vi "AIT 1553 - Clear Database.vi"(8 "error in (no error)":errorcluster, 11 "Node Ptr":u64 format="%.0x") -> (0 "error out":errorcluster)   [LabVIEW 2011, in "AIT 1553 Custom Device.lvlib"]
uses:
  AIT 1553 Custom Device.lvlib
  Controls and Global/Global.vi
  <vilib>/NI Veristand/Custom Device Tools/Custom Device Utility Library/NI VeriStand - Search for Item by GUID.vi
  <vilib>/NI Veristand/Custom Device API/Custom Device API.lvlib
  <vilib>/NI Veristand/Custom Device Tools/Custom Device Utility Library/Custom Device Utility Library.lvlib
panel:
  in  "Tag":string
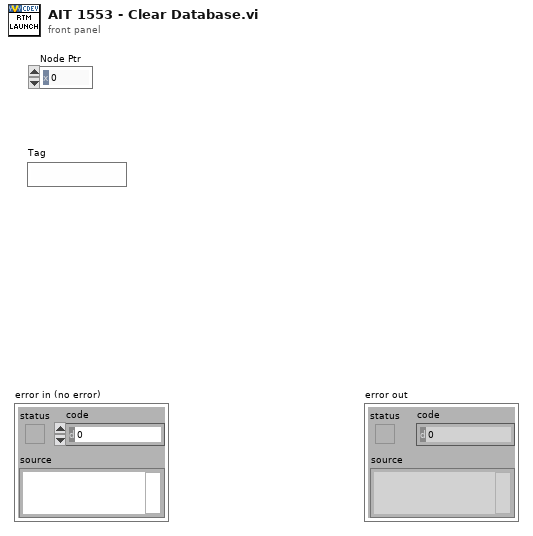
[diagram p1: front panel]
types:
  T1 = typedef "Custom Device API.lvlib/Custom Device Item Ref.ctl" = u64
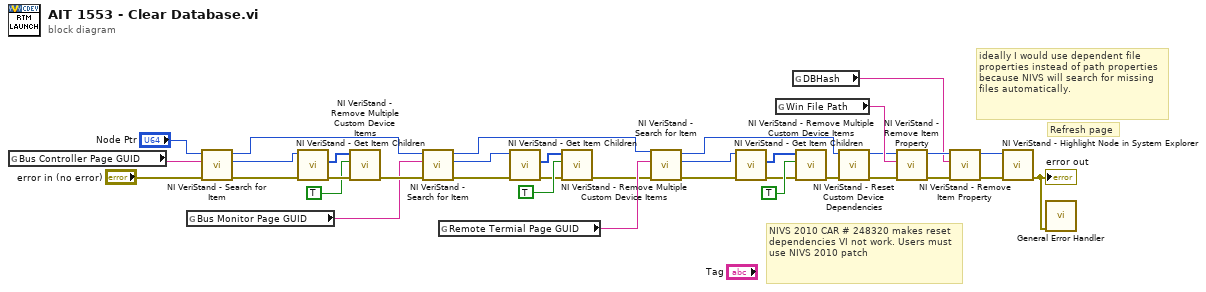
[diagram p0: block diagram]
diagram:
  # "ideally I would use dependent file properties instead of path properties because NIVS will search for missing files automatically."
  # "NIVS 2010 CAR # 248320 makes reset dependencies VI not work. Users must use NIVS 2010 patch"
  # "Refresh page"
  n1 = global read "Global.vi" "Bus Controller Page GUID"() -> (w29:string)
  n2 = global read "Global.vi" "Bus Monitor Page GUID"() -> (w1:string)
  n3 = call-poly <vilib>:"NI VeriStand - Search for Item.vi"("error in"="error in (no error)", "Item GUID"=w29, "Section Ref in"="Node Ptr") -> ("error out"=w24:errorcluster, "Item Ref"=w27:T1, "Section Ref out"=w9:T1)  [unwired: 5 in, 1 out]
  n4 = call <vilib>:"NI VeriStand - Get Item Children.vi"("error in (no error)"=w24, "Item Ref in"=w27) -> ("error out"=w35:errorcluster, "Child Refs"=w30:T1[])  [unwired: 6 in, 2 out]
  n5 = call <vilib>:"NI VeriStand - Remove Multiple Custom Device Items.vi"("error in (no error)"=w35, "Force Delete (F)"=TRUE, "Item Refs in"=w30) -> ("error out"=w10:errorcluster)  [unwired: 7 in, 1 out]
  n6 = call-poly <vilib>:"NI VeriStand - Search for Item.vi"("error in"=w10, "Item GUID"=w1, "Section Ref in"=w9) -> ("error out"=w4:errorcluster, "Item Ref"=w2:T1, "Section Ref out"=w8:T1)  [unwired: 5 in, 1 out]
  n7 = global read "Global.vi" "Remote Termial Page GUID"() -> (w11:string)
  n8 = call <vilib>:"NI VeriStand - Get Item Children.vi"("error in (no error)"=w4, "Item Ref in"=w2) -> ("error out"=w5:errorcluster, "Child Refs"=w7:T1[])  [unwired: 6 in, 2 out]
  n9 = call <vilib>:"NI VeriStand - Remove Multiple Custom Device Items.vi"("error in (no error)"=w5, "Force Delete (F)"=TRUE, "Item Refs in"=w7) -> ("error out"=w3:errorcluster)  [unwired: 7 in, 1 out]
  n10 = call-poly <vilib>:"NI VeriStand - Search for Item.vi"("error in"=w3, "Item GUID"=w11, "Section Ref in"=w8) -> ("error out"=w22:errorcluster, "Item Ref"=w23:T1, "Section Ref out"=w13:T1)  [unwired: 5 in, 1 out]
  n11 = call <vilib>:"NI VeriStand - Get Item Children.vi"("error in (no error)"=w22, "Item Ref in"=w23) -> ("error out"=w25:errorcluster, "Child Refs"=w12:T1[])  [unwired: 6 in, 2 out]
  n12 = global read "Global.vi" "Win File Path"() -> (w32:string)
  n13 = global read "Global.vi" "DBHash"() -> (w15:string)
  n14 = call <vilib>:"NI VeriStand - Remove Multiple Custom Device Items.vi"("error in (no error)"=w25, "Force Delete (F)"=TRUE, "Item Refs in"=w12) -> ("error out"=w21:errorcluster)  [unwired: 7 in, 1 out]
  n15 = call <vilib>:"NI VeriStand - Reset Custom Device Dependencies.vi"("error in (no error)"=w21, "Device Ref in"=w13) -> ("error out"=w33:errorcluster, "Device Ref out"=w31:T1)  [unwired: 8 in]
  n16 = call <vilib>:"NI VeriStand - Remove Item Property.vi"("error in (no error)"=w33, "Property Name"=w32, "Item Ref in"=w31) -> ("error out"=w19:errorcluster, "Item Ref out"=w18:T1)  [unwired: 6 in, 1 out]
  n17 = call <vilib>:"NI VeriStand - Remove Item Property.vi"("error in (no error)"=w19, "Property Name"=w15, "Item Ref in"=w18) -> ("error out"=w17:errorcluster, "Item Ref out"=w16:T1)  [unwired: 6 in, 1 out]
  n18 = call <vilib>:"NI VeriStand - Highlight Node in System Explorer.vi"("error in (no error)"=w17, "Item Ref in"=w16) -> ("error out"=w20:errorcluster)  [unwired: 8 in, 1 out]
  "error out" <- w20
  n19 = call <vilib>:"General Error Handler.vi"("error in (no error)"=w20) -> ()  [unwired: 10 in, 5 out]
